vi "Close.vi"(8 "error in (no error)":errorcluster, 11 "VGC in":refnum<class "PL Inficon VGC.lvclass">) -> (0 "error out":errorcluster)   [LabVIEW 2015, in "PL Inficon VGC.lvclass"]
doc: "Closes connection to device."
uses:
  PL Inficon VGC.lvclass
  PL Inficon VGC.lvclass/PL Inficon VGC.ctl
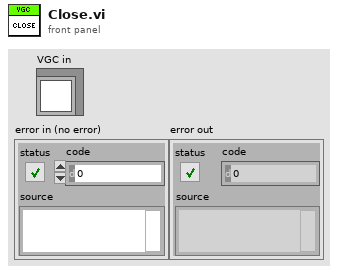
[diagram p1: front panel]
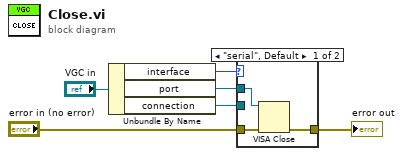
[diagram p0: block diagram]
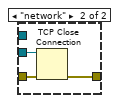
[diagram p2: hidden frame]
diagram:
  n1 = Unbundle By Name("VGC in") -> ("interface"=w1:enum16{"serial", "network"}, "port"=w5:refnum<visa-resource-name>, "connection"=w2:refnum<k5>)
  n2 = case shown="\"serial\", Default" w1 {
    tunnel: w5 -> [w9 _]
    tunnel: "error in (no error)" -> [w8 w11]
    tunnel: [w7 w10] -> w3
    tunnel: w2 -> [_ w12]
    frame "serial", Default {
      n3 = VISA Close(VISA resource name=w9, error in (no error)=w8) -> (error out=w7:errorcluster)
    }
    frame "network" {
      n4 = TCP Close Connection(connection ID=w12, error in (no error)=w11) -> (error out=w10:errorcluster)  [unwired: 1 in, 1 out]
    }
  }
  "error out" <- w3
